vi "detect network devices.vi"(4 "remote timeout (300,000 ms)":u32=300000, 6 "detect all (F)":bool, 7 "local subnet only (F)":bool, 8 "error in":errorcluster, 10 "device class":T2, 11 "system session (localhost)":refnum<k21>="localhost") -> (0 "error out":errorcluster, 2 "devices":T1[](array[typedef]) {"product ID" format="%.0x"}, 3 "system session out":refnum<k21>)   [LabVIEW 2013, in "SMI.lvlib" / "Device.lvclass"]
uses:
  Device.lvclass
  device class selection.ctl
  network device information.ctl
  <vilib>/nisyscfg/Filter Mode.ctl
  <vilib>/nisyscfg/Close (Filter).vi
  <vilib>/nisyscfg/Close (Resources).vi
  <vilib>/regexp/Match Regular Expression.xnode
  <vilib>/nisyscfg/nisyscfg.lvlib
  <resource>/objmgr/nisysapi.rc
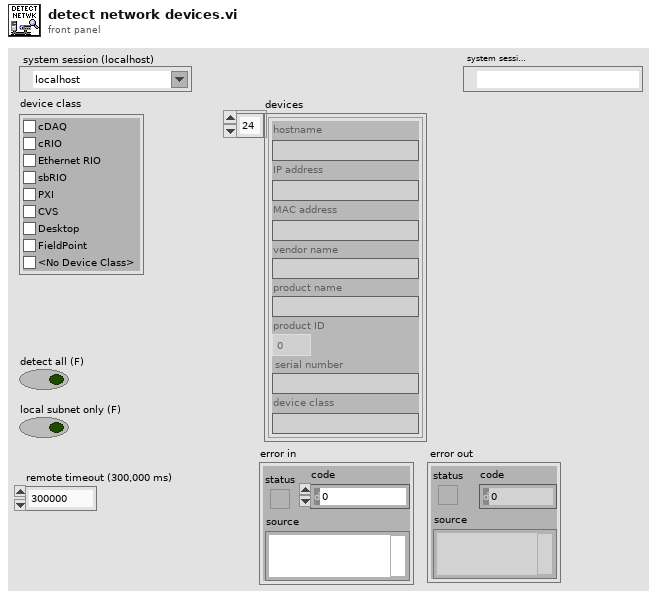
[diagram p1: front panel]
types:
  T1 = typedef "SMI.lvlib/Device.lvclass/network device information.ctl" = cluster{"hostname":string, "IP address":string, "MAC address":string, "vendor name":string, "product name":string, "product ID":u16, "serial number":string, "device class":string}
  T2 = typedef "SMI.lvlib/Device.lvclass/device class selection.ctl" = cluster{"cDAQ":bool, "cRIO":bool, "Ethernet RIO":bool, "sbRIO":bool, "PXI":bool, "CVS":bool, "Desktop":bool, "FieldPoint":bool, "<No Device Class>":bool}
  T3 = typedef "nisyscfg.lvlib/Filter Mode.ctl" = i32
  T4 = typedef "SMI.lvlib/Device.lvclass/device class.ctl" = enum16{"cDAQ", "cRIO", "Ethernet RIO", "sbRIO", "PXI", "CVS", "Desktop", "FieldPoint", "<No Device Class>", "<Detect All>"}
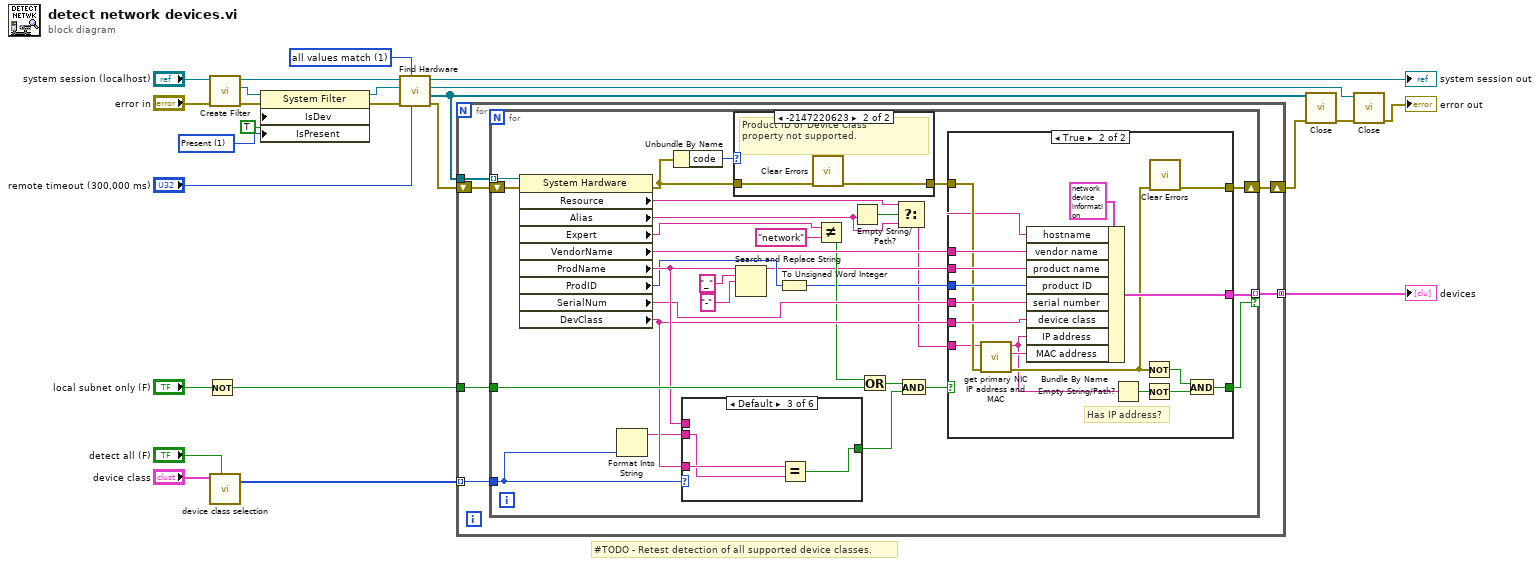
[diagram p0: block diagram]
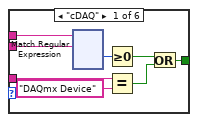
[diagram p4: hidden frame]
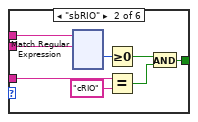
[diagram p5: hidden frame]
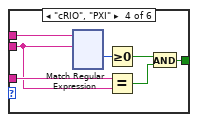
[diagram p6: hidden frame]
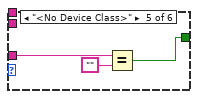
[diagram p7: hidden frame]
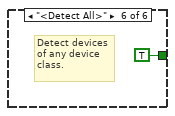
[diagram p8: hidden frame]
diagram:
  w4 = 1 items=["Initializing"=-2, "Unknown"=-1, "Not Present"=0, "Present"=1] ("Devices & Chassis:Is Present")
  w15 = T3 1 items=["all values match"=1, "any value matches"=2, "values do not match"=3, "all properties exist"=4] ("filter mode (all values match)")
  # "#TODO - Retest detection of all supported device classes."
  n1 = Not(x="local subnet only (F)") -> (.not. x?=w21:bool)
  n2 = call <vilib>:"Create Filter.vi"("error in (no error)"="error in", "Session in"="system session (localhost)") -> ("error out"=w20:errorcluster, "Filter out"=w19:refnum<k20>, "Session out"=w18:refnum<k21>)  [unwired: 7 in]
  n3 = call "device class selection.vi"("detect all (F)"="detect all (F)", "device classes"="device class") -> ("device class"=w1:T4[])  [unwired: 5 in]
  n4 = property class="System Filter"(reference=w19, error in=w20, "IsDev"=TRUE ("Is Chassis"), "IsPresent"=w4) -> (reference out=w16:refnum<k20>, error out=w17:errorcluster)
  n5 = call <vilib>:"Find Hardware.vi"("Remote Timeout (300,000 ms)"="remote timeout (300,000 ms)", "Filter Mode (all values match)"=w15, "error in (no error)"=w17, "Filter in"=w16, "Session in"=w18) -> ("error out"=w14:errorcluster, "Resources out"=w13:refnum<k20>[], "Filter out"=w11:refnum<k20>, "Session out"=→"system session out":refnum<k21>)  [unwired: 3 out]
  n6 = for {
    tunnel: w21 -> [w30]
    tunnel: w13 -> [w28]
    tunnel: w1 -> [w26] mode=indexing
    shift-right: [w27] -> w10
    shift-left: w14 -> [w29]
    tunnel: [w25] -> w3 mode=concatenating
    n7 = for {
      tunnel: w28 -> [w60] mode=indexing
      shift-right: [w54] -> w27
      shift-left: w29 -> [w59]
      tunnel: w30 -> [w58]
      tunnel: w26 -> [w32]
      tunnel: [w40] -> w25 mode=indexing if=w35
      n8 = property class="System Hardware"(reference=w60, error in=w59) -> (error out=w34:errorcluster, "Resource"=w39:string, "Alias"=w57:string, "Expert"=w56:string, "VendorName"=w55:string, "ProdName"=w53:string, "ProdID"=w50:u32, "SerialNum"=w51:string, "DevClass"=w52:string)  [unwired: 1 out]
      n9 = Format Into String(w32) -> (resulting string=w31:string)  [unwired: 3 in, 1 out]
      n10 = Unbundle By Name(w34) -> ("code"=w33:i32)
      n11 = case shown="Default" w32 {
        tunnel: w52 -> [w89 w211 w329 w335 w453 _]
        tunnel: w53 -> [w90 w212 _ w336 _ _]
        tunnel: [w85 w207 w328 w331 w452 TRUE] -> w46
        tunnel: w31 -> [w83 w205 w327 w330 _ _]
        frame "cDAQ" {
          n12 = xnode "Match Regular Expression"("input string"=w90, "regular expression"=w83) -> ("offset past match"=w88:i32)  [unwired: 4 in, 4 out]
          n13 = Greater Or Equal To 0?(x=w88) -> (x >= 0?=w86:bool)
          n14 = Equal?(x=w89, y="DAQmx Device") -> (x = y?=w87:bool)
          n15 = Or(x=w86, y=w87) -> (x .or. y?=w85:bool)
        }
        frame "sbRIO" {
          n16 = xnode "Match Regular Expression"("input string"=w212, "regular expression"=w205) -> ("offset past match"=w210:i32)  [unwired: 4 in, 4 out]
          n17 = Greater Or Equal To 0?(x=w210) -> (x >= 0?=w208:bool)
          n18 = Equal?(x=w211, y="cRIO") -> (x = y?=w209:bool)
          n19 = And(x=w208, y=w209) -> (x .and. y?=w207:bool)
        }
        frame Default {
          n20 = Equal?(x=w329, y=w327) -> (x = y?=w328:bool)
        }
        frame "cRIO", "PXI" {
          n21 = xnode "Match Regular Expression"("input string"=w336, "regular expression"=w330) -> ("offset past match"=w334:i32)  [unwired: 4 in, 4 out]
          n22 = Greater Or Equal To 0?(x=w334) -> (x >= 0?=w332:bool)
          n23 = Equal?(x=w335, y=w330) -> (x = y?=w333:bool)
          n24 = And(x=w332, y=w333) -> (x .and. y?=w331:bool)
        }
        frame "<No Device Class>" {
          n25 = Equal?(x=w453, y="") -> (x = y?=w452:bool)
        }
        frame "<Detect All>" {
          # "Detect devices\nof any device\nclass."
        }
      }
      n26 = case shown="-2147220623" w33 {
        tunnel: w34 -> [w61 w63]
        tunnel: [w61 w62] -> w38
        frame 0, Default {
        }
        frame -2147220623 {
          # "Product ID or Device Class\nproperty not supported."
          n27 = call <vilib>:"Clear Errors.vi"("error in (no error)"=w63) -> ("error out"=w62:errorcluster)  [unwired: 6 in]
        }
      }
      n28 = Search and Replace String(input string=w53, search string="_", replace string="-" ("replace string (\"\")")) -> (result string=w42:string)  [unwired: 5 in, 3 out]
      n29 = To Unsigned Word Integer(number=w50) -> (unsigned 16bit integer=w41:u16)
      n30 = Not Equal?(x=w56, y="network") -> (x != y?=w47:bool)
      n31 = Empty String/Path?(string/path=w57) -> (empty?=w49:bool)
      n32 = Or(x=w47, y=w58) -> (x .or. y?=w45:bool)
      n33 = Select(t=w39, s=w49, f=w57) -> (s? t:f=w37:string)
      n34 = And(x=w45, y=w46) -> (x .and. y?=w36:bool)
      n35 = case shown="True" w36 {
        selector: w36 -> [w64 _]
        tunnel: w55 -> [_ w82]
        tunnel: [w65 w81] -> w54
        tunnel: w52 -> [_ w80]
        tunnel: w51 -> [_ w79]
        tunnel: w42 -> [_ w77]
        tunnel: w41 -> [_ w76]
        tunnel: [_ w75] -> w40
        tunnel: w38 -> [w65 w73]
        tunnel: w37 -> [_ w71]
        tunnel: [w64 w66] -> w35
        frame False {
        }
        frame True {
          # "Has IP address?"
          n36 = call "get primary NIC IP address and MAC.vi"("error in"=w73, "system session"=w71) -> ("error out"=w72:errorcluster, "MAC address"=w74:string, "IP address"=w69:string)  [unwired: 7 in]
          n37 = Bundle By Name(cluster=T1 {"hostname"="cRIO-9014-Test", "IP address"="", "MAC address"="", "vendor name"="National Instruments", "product name"="", "product ID"=29071, "serial number"="00E86EAB", "device class"=""} ("Device Information"), "hostname"=w71, "vendor name"=w82, "product name"=w77, "product ID"=w76, "serial number"=w79, "device class"=w80, "IP address"=w69, "MAC address"=w74) -> (w75:T1)
          n38 = Empty String/Path?(string/path=w69) -> (empty?=w70:bool)
          n39 = Not(x=w72) -> (.not. x?=w67:bool)
          n40 = Not(x=w70) -> (.not. x?=w68:bool)
          n41 = call <vilib>:"Clear Errors.vi"("error in (no error)"=w72) -> ("error out"=w81:errorcluster)  [unwired: 6 in]
          n42 = And(x=w67, y=w68) -> (x .and. y?=w66:bool)
        }
      }
    }
  }
  "devices" <- w3
  n43 = call-poly <vilib>:"Close.vi"("error in (no error)"=w10, "Resources in"=w13) -> ("error out"=w9:errorcluster)  [unwired: 9 in]
  n44 = call-poly <vilib>:"Close.vi"("error in (no error)"=w9, "Filter in"=w11) -> ("error out"=→"error out":errorcluster)  [unwired: 9 in]
